vi "CTRE_CANifier_SetGeneralOutputs.vi"(8 "error in":errorcluster, 9 "Is Output?":T1={"QUAD_IDX"=TRUE, "QUAD_B"=TRUE, "QUAD_A"=TRUE, "LIMR"=TRUE, "LIMF"=TRUE, "SDA"=TRUE, "SCL"=TRUE, "SPI_CS"=TRUE, "SPI_MISO_PWM2"=TRUE, "SPI_MOSI_PWM1"=TRUE, "SPI_CLK_PWM0"=TRUE}, 10 "Output State":T1={"QUAD_IDX"=TRUE, "QUAD_B"=TRUE, "QUAD_A"=TRUE, "LIMR"=TRUE, "LIMF"=TRUE, "SDA"=TRUE, "SCL"=TRUE, "SPI_CS"=TRUE, "SPI_MISO_PWM2"=TRUE, "SPI_MOSI_PWM1"=TRUE, "SPI_CLK_PWM0"=TRUE}, 11 "CANifierDevRef":T2) -> (0 "error out":errorcluster, 3 "CANifierDevRef":T2)   [LabVIEW 2019]
uses:
  <vilib>/Rock Robotics/WPI/ThirdParty/Phoenix-LabVIEW/CANifier/CTRE_CANifier_DeviceRef.ctl
  <vilib>/Rock Robotics/WPI/ThirdParty/Phoenix-LabVIEW/CANifier/CTRE_CANifier_GeneralPinsCluster.ctl
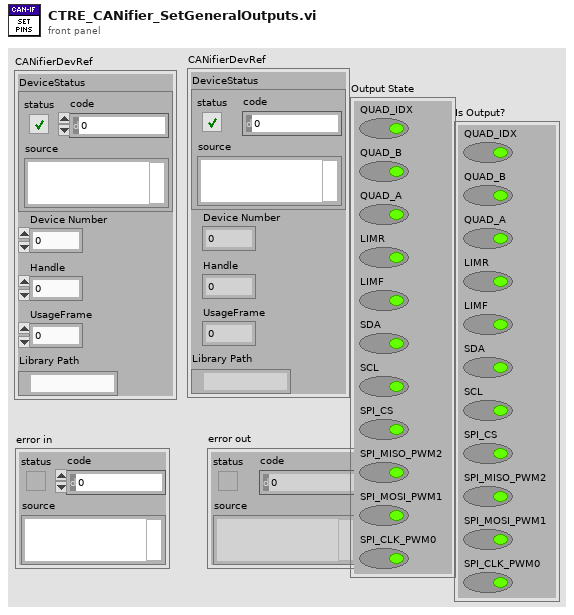
[diagram p1: front panel]
types:
  T1 = typedef "CTRE_CANifier_GeneralPinsCluster.ctl" = cluster{"QUAD_IDX":bool, "QUAD_B":bool, "QUAD_A":bool, "LIMR":bool, "LIMF":bool, "SDA":bool, "SCL":bool, "SPI_CS":bool, "SPI_MISO_PWM2":bool, "SPI_MOSI_PWM1":bool, "SPI_CLK_PWM0":bool}
  T2 = typedef "CTRE_CANifier_DeviceRef.ctl" = cluster{"DeviceStatus":errorcluster, "Device Number":u8, "Handle":u64, "UsageFrame":u32, "Library Path":path}
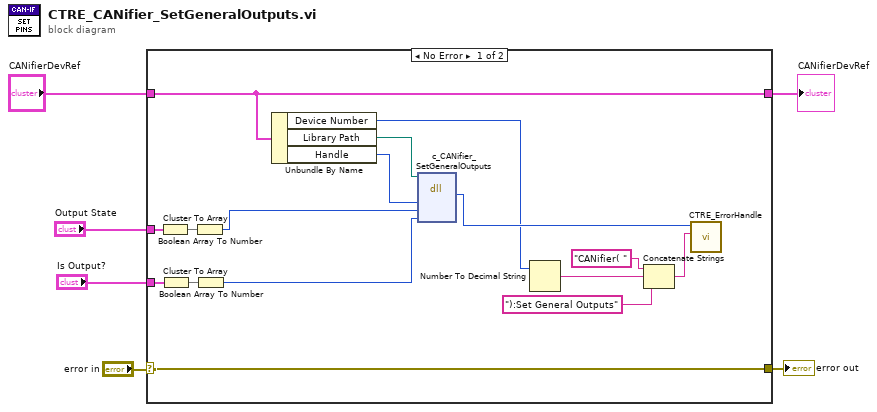
[diagram p0: block diagram]
diagram:
  n1 = case shown="No Error" "error in" {
    selector: "error in" -> [w22 w24]
    tunnel: [w22 w24] -> w5
    tunnel: "CANifierDevRef" -> [w21 w23]
    tunnel: [w21 w23] -> w3
    tunnel: "Output State" -> [w12 _]
    tunnel: "Is Output?" -> [w9 _]
    frame No Error {
      n2 = Cluster To Array(cluster=w12) -> (array=w11:bool[])
      n3 = Cluster To Array(cluster=w9) -> (array=w10:bool[])
      n4 = Boolean Array To Number(Boolean array=w11) -> (number=w8:u32)
      n5 = Boolean Array To Number(Boolean array=w10) -> (number=w7:u32)
      n6 = Unbundle By Name(w21) -> ("Device Number"=w14:u8, "Library Path"=w20:path, "Handle"=w19:u64)
      n7 = dll-call lib="?" fn="c_CANifier_SetGeneralOutputs"(path in=w20, "handle"=w19, "outputBits"=w8, "isOutputBits"=w7) -> ("CTR_Code"=w18:i8)  [unwired: 5 in, 2 out]
      n8 = Number To Decimal String(number=w14) -> (decimal integer string=w17:string)  [unwired: 1 in]
      n9 = Concatenate Strings("CANifier( " ("string"), w17, "):Set General Outputs" ("string")) -> (w13:string)
      n10 = call <vilib>:"CTRE_ErrorHandle.vi"("origin"=w13, "code"=w18) -> ()  [unwired: 9 in, 1 out]
    }
    frame Error {
    }
  }
  "error out" <- w5
  "CANifierDevRef" <- w3
